vi "DriveGetGyroCalibrated.vi"() -> (3 "GryoCalibrated":bool)   [LabVIEW 2020]
doc: "Put drive global variable Gyro X into Pitch to use in other VI's\n\nOutputs:\n-- Pitch -- Double -- Pitch of the robot (back and forth angle) --"
uses:
  DriveGlobal.vi
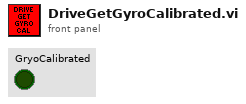
[diagram p1: front panel]
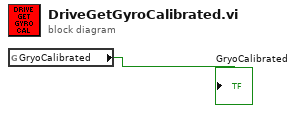
[diagram p0: block diagram]
diagram:
  n1 = global read "DriveGlobal.vi" "GryoCalibrated"() -> (→"GryoCalibrated":bool)
